vi "Autonomous Independent.vi"   [LabVIEW 2015]
doc: "This VI is called when autonomous begins, and will automatically be terminated when autonomous ends. You can carry out timed or sensor driven robot movement independently without needing to return to the caller."
uses:
  <vilib>/Rock Robotics/WPI/Utilities/WPI_GetSetVariantRefNum.vi
  <vilib>/Rock Robotics/Network Tables/NT Read String.vi
  <vilib>/Rock Robotics/Network Tables/NT Write Numeric Array.vi
panel:
  # "Be sure to right-click and choose Data Operations>>Make Current Value default if you want to save the array values with the VI"
types:
  T1 = typedef "WPI_JoystickDevRef.ctl" = cluster{"Device":T2}
  T2 = typedef "WPI_JoystickDeviceEnum.ctl" = enum16{"USB 0", "USB 1", "USB 2", "USB 3", "USB 4", "USB 5"}
  T3 = typedef "WPI_ServoDeviceRef.ctl" = cluster{"DeviceStatus":errorcluster, "PWM Channel":T4, "DeadBand":T5}
  T4 = typedef "FPGA_DIOPWMChannel.ctl" = enum8{"PWM 0", "PWM 1", "PWM 2", "PWM 3", "PWM 4", "PWM 5", "PWM 6", "PWM 7", "PWM 8", "PWM 9", "PWM MXP 0", "PWM MXP 1", "PWM MXP 2", "PWM MXP 3", "PWM MXP 4", "PWM MXP 5", "PWM MXP 6", "PWM MXP 7", "PWM MXP 8", "PWM MXP 9", "Invalid"}
  T5 = typedef "WPI_PWMDeadband.ctl" = cluster{"Name":string, "maxPositivePwm":i32, "minPositivePwm":i32, "centerPwm":i32, "maxNegativePwm":i32, "minNegativePwm":i32, "angularRange":u16}
  T6 = typedef "WPI_DigitalInputDevRef.ctl" = cluster{"DevStatus":errorcluster, "DIO Channel":T7}
  T7 = typedef "FPGA_DIOChannel.ctl" = enum8{"DIO 0", "DIO 1", "DIO 2", "DIO 3", "DIO 4", "DIO 5", "DIO 6", "DIO 7", "DIO 8", "DIO 9", "DIO MXP 0", "DIO MXP 1", "DIO MXP 2", "DIO MXP 3", "DIO MXP 4", "DIO MXP 5", "DIO MXP 6", "DIO MXP 7", "DIO MXP 8", "DIO MXP 9", "DIO MXP 10", "DIO MXP 11", "DIO MXP 12", "DIO MXP 13", "DIO MXP 14", "DIO MXP 15", "Invalid"}
  T8 = typedef "WPI_MotorControlDeviceRef.ctl" = cluster{"DeviceStatus":errorcluster, "Type":T9, "PWM":cluster{"PWM Channel":T4, "DeadBand":T5}, "CAN":cluster{"Device Number":u8, "Control Mode":T10, "Semaphore":T11, "Max Vout":dbl, "TalonSRX Control Mode":T12}, "Invert":bool}
  T9 = typedef "WPI_MotorControlType.ctl" = enum16{"PWM", "CAN", "CANTalonSRX"}
  T10 = typedef "WPI_CANJaguar_ControlMode.ctl" = enum8{"Percent VBus", "Current", "Speed", "Position", "Voltage"}
  T11 = typedef "Semaphore RefNum" = refnum<k1>
  T12 = typedef "WPI_CANTalonSRX_APIControlMode.ctl" = enum8{"Percent VBus", "Speed", "Position", "Slave", "Unchanged / Invalid", "Voltage Compensation", "Current", "Motion Profile"}
  T13 = typedef "WPI_RobotDriveDevRef.ctl" = cluster{"DevStatus":errorcluster, "Motors[]":T8[], "Square Inputs":bool, "Max Output":dbl}
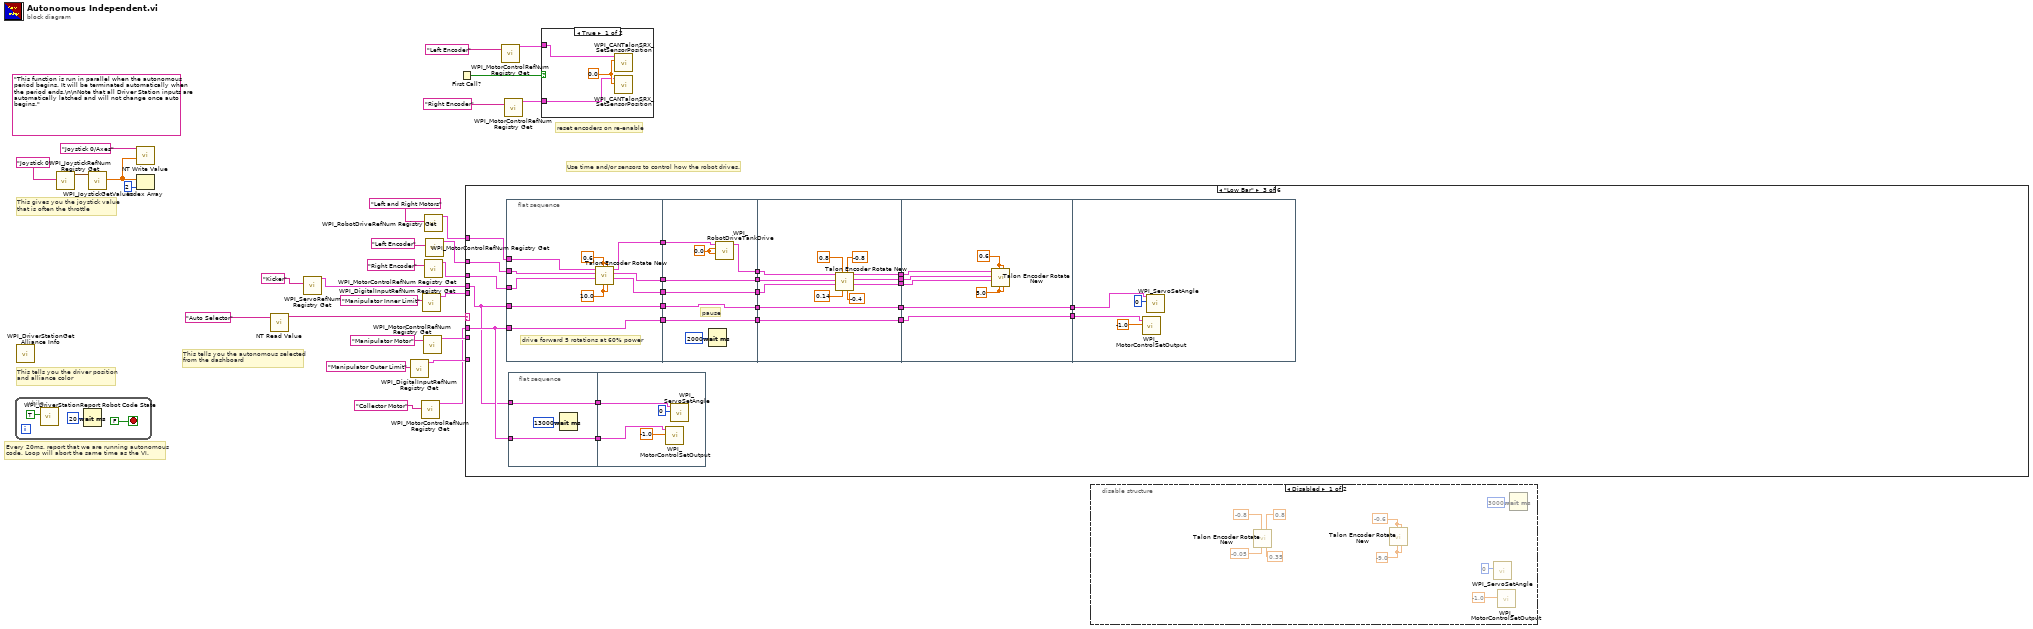
[diagram p0: block diagram]
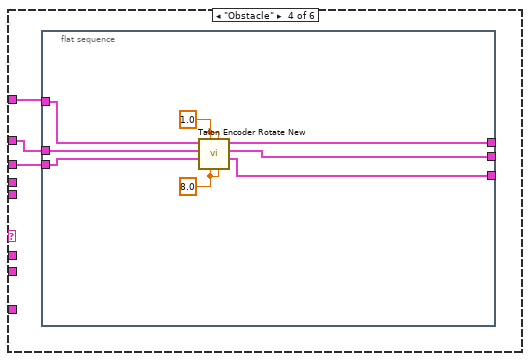
[diagram p6: hidden frame]
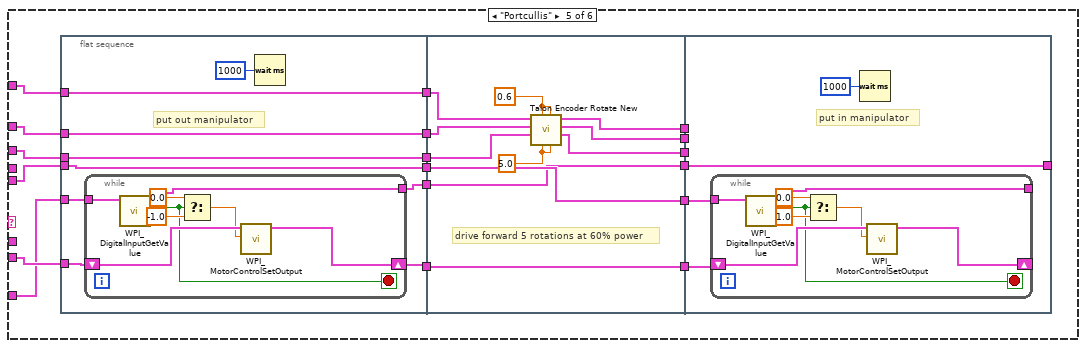
[diagram p7: hidden frame]
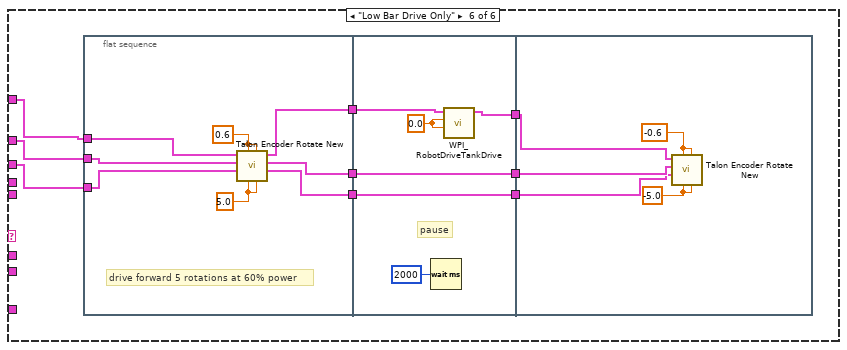
[diagram p8: hidden frame]
diagram:
  (unwired) "This function is run in parallel when the autonomous period begins. It will be terminated automatically when the period ends.\n\nNote that all Driver Station inputs are automatically latched and will not change once auto begins."
  # "reset encoders on re-enable"
  # "This tells you the autonomous selected\nfrom the dashboard"
  # "Every 20ms, report that we are running autonomous\ncode. Loop will abort the same time as the VI."
  # "This gives you the joystick value\nthat is often the throttle"
  # "Use time and/or sensors to control how the robot drives."
  # "This tells you the driver position\nand alliance color"
  n1 = while {
    stop <- FALSE stop-if-true
    n2 = call <vilib>:"WPI_DriverStationReport Robot Code State.vi"("Autonomous"=TRUE) -> ()  [unwired: 10 in, 1 out]
    n3 = Wait (ms)(milliseconds to wait=u32 20) -> ()  [unwired: 1 out]
  }
  n4 = call <vilib>:"WPI_DriverStationGet Alliance Info.vi"() -> ()  [unwired: 12 out]
  n5 = call <vilib>:"WPI_JoystickRefNum Registry Get.vi"("refnum name"="Joystick 0") -> ("JoystickDevRef"=w27:T1)  [unwired: 1 in, 9 out]
  n6 = call <vilib>:"WPI_JoystickGetValues.vi"("JoystickDevRef"=w27) -> ("Axes"=w23:dbl[])  [unwired: 6 in, 4 out]
  n7 = call-poly <vilib>:"NT Write Value.vi"("Numeric Array"=w23, "Name"="Joystick 0/Axes") -> ()  [unwired: 9 in, 1 out]
  n8 = Index Array(array=w23, index=2) -> ()  [unwired: 1 out]
  n9 = call-poly <vilib>:"NT Read Value.vi"("Name"="Auto Selector") -> ("String"=w24:string)  [unwired: 9 in, 1 out]
  n10 = call <vilib>:"WPI_ServoRefNum Registry Get.vi"("refnum name"="Kicker") -> ("ServoDeviceRef"=w1:T3)  [unwired: 9 in, 1 out]
  n11 = call <vilib>:"WPI_DigitalInputRefNum Registry Get.vi"("refnum name"="Manipulator Outer Limit") -> ("DigitalInputDevRef"=w7:T6)  [unwired: 9 in, 1 out]
  n12 = call <vilib>:"WPI_MotorControlRefNum Registry Get.vi"("refnum name"="Collector Motor") -> ("MotorControlDevRef"=w3:T8)  [unwired: 9 in, 1 out]
  n13 = call <vilib>:"WPI_DigitalInputRefNum Registry Get.vi"("refnum name"="Manipulator Inner Limit") -> ("DigitalInputDevRef"=w5:T6)  [unwired: 9 in, 1 out]
  n14 = call <vilib>:"WPI_MotorControlRefNum Registry Get.vi"("refnum name"="Manipulator Motor") -> ("MotorControlDevRef"=w9:T8)  [unwired: 9 in, 1 out]
  n15 = call <vilib>:"WPI_RobotDriveRefNum Registry Get.vi"("refnum name"="Left and Right Motors") -> ("RobotDriveDevRef"=w13:T13)  [unwired: 1 in, 9 out]
  n16 = call <vilib>:"WPI_MotorControlRefNum Registry Get.vi"("refnum name"="Right Encoder") -> ("MotorControlDevRef"=w12:T8)  [unwired: 9 in, 1 out]
  n17 = call <vilib>:"WPI_MotorControlRefNum Registry Get.vi"("refnum name"="Left Encoder") -> ("MotorControlDevRef"=w11:T8)  [unwired: 9 in, 1 out]
  n18 = First Call?() -> (First Call?: T/F=w21:bool)
  n19 = case shown="\"Low Bar\"" w24 {
    tunnel: w13 -> [_ _ w55 w106 w132 w178]
    tunnel: w12 -> [_ _ w53 w104 w130 w176]
    tunnel: w11 -> [_ _ w54 w105 w131 w177]
    tunnel: w9 -> [_ _ _ _ w129 _]
    tunnel: w7 -> [_ _ _ _ w128 _]
    tunnel: w5 -> [_ _ _ _ w123 _]
    tunnel: w3 -> [_ _ w34 _ _ _]
    tunnel: w1 -> [_ _ w32 _ _ _]
    frame "None", Default {
    }
    frame "Teeter Totter" {
    }
    frame "Low Bar" {
      n20 = flat-sequence {
        tunnel: w55 -> [w72]
        tunnel: w54 -> [w71]
        tunnel: w53 -> [w70]
        tunnel: [w69] -> w51
        tunnel: [w66] -> w49
        tunnel: [w65] -> w47
        tunnel: [w64] -> w41
        tunnel: w34 -> [w64]
        tunnel: w32 -> [w63]
        tunnel: [w63] -> w38
        tunnel: [w80] -> w52
        tunnel: w51 -> [w77]
        tunnel: [w76] -> w50
        tunnel: w49 -> [w76]
        tunnel: [w75] -> w48
        tunnel: w47 -> [w75]
        tunnel: [w74] -> w42
        tunnel: w41 -> [w74]
        tunnel: [w73] -> w39
        tunnel: w38 -> [w73]
        tunnel: w52 -> [w92]
        tunnel: w50 -> [w91]
        tunnel: w48 -> [w90]
        tunnel: [w89] -> w46
        tunnel: [w88] -> w45
        tunnel: [w87] -> w44
        tunnel: [w82] -> w43
        tunnel: w42 -> [w82]
        tunnel: [w81] -> w40
        tunnel: w39 -> [w81]
        tunnel: w46 -> [w98]
        tunnel: w45 -> [w97]
        tunnel: w44 -> [w96]
        tunnel: w43 -> [w93]
        tunnel: w40 -> [w94]
        tunnel: [w94] -> w37
        tunnel: [w93] -> w36
        tunnel: w37 -> [w101]
        tunnel: w36 -> [w100]
        frame #0 {
          w67 = 10.0 ("Rotations")
          w68 = 0.6 ("Speed")
          # "drive forward 5 rotations at 60% power"
          n21 = call "Talon Encoder Rotate New.vi"("Right Rotations"=w67, "Right Speed"=w68, "Left Rotations"=w67, "Left Speed"=w68, "RightEncoderMotorRef"=w70, "LeftEncoderMotorRef"=w71, "RobotDriveDevRef"=w72) -> ("RightEncoderMotorRef"=w65:T8, "LeftEncoderMotorRef"=w66:T8, "RobotDriveDevRef"=w69:T13)  [unwired: 2 in]
        }
        frame #1 {
          w79 = 0.0 ("Left axis value")
          # "pause"
          n22 = Wait (ms)(milliseconds to wait=u32 2000) -> ()  [unwired: 1 out]
          n23 = call <vilib>:"WPI_RobotDriveTankDrive.vi"("Right axis value"=w79, "Left axis value"=w79, "RobotDriveDevRef"=w77) -> ("RobotDriveDevRef"=w80:T13)  [unwired: 6 in, 2 out]
        }
        frame #2 {
          n24 = call "Talon Encoder Rotate New.vi"("Right Rotations"=-0.4, "Right Speed"=-0.8, "Left Rotations"=0.14, "Left Speed"=0.8, "RightEncoderMotorRef"=w90, "LeftEncoderMotorRef"=w91, "RobotDriveDevRef"=w92) -> ("RightEncoderMotorRef"=w87:T8, "LeftEncoderMotorRef"=w88:T8, "RobotDriveDevRef"=w89:T13)  [unwired: 2 in]
        }
        frame #3 {
          w95 = 5.0 ("Left Rotations")
          w99 = 0.6 ("Speed")
          n25 = call "Talon Encoder Rotate New.vi"("Right Rotations"=w95, "Right Speed"=w99, "Left Rotations"=w95, "Left Speed"=w99, "RightEncoderMotorRef"=w96, "LeftEncoderMotorRef"=w97, "RobotDriveDevRef"=w98) -> ()  [unwired: 2 in, 3 out]
        }
        frame #4 {
          n26 = call <vilib>:"WPI_MotorControlSetOutput.vi"("Output"=-1.0, "MotorControlDevRef"=w100) -> ()  [unwired: 7 in, 3 out]
          n27 = call <vilib>:"WPI_ServoSetAngle.vi"("Angle"=0, "ServoDeviceRef"=w101) -> ()  [unwired: 8 in, 2 out]
        }
      }
      n28 = flat-sequence {
        tunnel: [w57] -> w35
        tunnel: w34 -> [w57]
        tunnel: [w56] -> w33
        tunnel: w32 -> [w56]
        tunnel: w35 -> [w60]
        tunnel: w33 -> [w59]
        frame #0 {
          n29 = Wait (ms)(milliseconds to wait=u32 13000) -> ()  [unwired: 1 out]
        }
        frame #1 {
          n30 = call <vilib>:"WPI_MotorControlSetOutput.vi"("Output"=-1.0, "MotorControlDevRef"=w60) -> ()  [unwired: 7 in, 3 out]
          n31 = call <vilib>:"WPI_ServoSetAngle.vi"("Angle"=0, "ServoDeviceRef"=w59) -> ()  [unwired: 8 in, 2 out]
        }
      }
    }
    frame "Obstacle" {
      n32 = flat-sequence {
        tunnel: w106 -> [w114]
        tunnel: w105 -> [w113]
        tunnel: w104 -> [w112]
        tunnel: [w109] -> _
        tunnel: [w108] -> _
        tunnel: [w107] -> _
        frame #0 {
          w110 = 8.0 ("Rotations")
          w111 = 1.0 ("Speed")
          n33 = call "Talon Encoder Rotate New.vi"("Right Rotations"=w110, "Right Speed"=w111, "Left Rotations"=w110, "Left Speed"=w111, "RightEncoderMotorRef"=w112, "LeftEncoderMotorRef"=w113, "RobotDriveDevRef"=w114) -> ("RightEncoderMotorRef"=w107:T8, "LeftEncoderMotorRef"=w108:T8, "RobotDriveDevRef"=w109:T13)  [unwired: 2 in]
        }
      }
    }
    frame "Portcullis" {
      n34 = flat-sequence {
        tunnel: w129 -> [w138]
        tunnel: w132 -> [w139]
        tunnel: w130 -> [w140]
        tunnel: w131 -> [w141]
        tunnel: [w141] -> w120
        tunnel: [w140] -> w119
        tunnel: [w139] -> w118
        tunnel: [w137] -> w117
        tunnel: w128 -> [w136]
        tunnel: w123 -> [w134]
        tunnel: [w134] -> w116
        tunnel: [w133] -> w115
        tunnel: w120 -> [w158]
        tunnel: w119 -> [w157]
        tunnel: w118 -> [w159]
        tunnel: w117 -> [w160]
        tunnel: [w160] -> w127
        tunnel: [w154] -> w126
        tunnel: [w153] -> w125
        tunnel: [w152] -> w124
        tunnel: [w151] -> w122
        tunnel: w116 -> [w151]
        tunnel: w115 -> [w150]
        tunnel: [w150] -> w121
        tunnel: w127 -> [w164]
        tunnel: w126 -> [_]
        tunnel: w125 -> [_]
        tunnel: w124 -> [_]
        tunnel: w122 -> [w163]
        tunnel: w121 -> [w161]
        tunnel: [w161] -> _
        frame #0 {
          # "put out manipulator"
          n35 = while {
            shift-right: [w148] -> w137
            shift-left: w138 -> [w149]
            tunnel: w136 -> [w147]
            tunnel: [w142] -> w133
            stop <- w143 stop-if-true
            n36 = call <vilib>:"WPI_DigitalInputGetValue.vi"("DigitalInputDevRef"=w147) -> ("Value"=w143:bool, "DigitalInputDevRef"=w142:T6)  [unwired: 8 in, 1 out]
            n37 = Select(t=0.0, s=w143, f=-1.0) -> (s? t:f=w144:dbl)
            n38 = call <vilib>:"WPI_MotorControlSetOutput.vi"("Output"=w144, "MotorControlDevRef"=w149) -> ("MotorControlDevRef"=w148:T8)  [unwired: 7 in, 2 out]
          }
          n39 = Wait (ms)(milliseconds to wait=u32 1000) -> ()  [unwired: 1 out]
        }
        frame #1 {
          w156 = 5.0 ("Left Rotationos")
          w155 = 0.6 ("Speed")
          # "drive forward 5 rotations at 60% power"
          n40 = call "Talon Encoder Rotate New.vi"("Right Rotations"=w156, "Right Speed"=w155, "Left Rotations"=w156, "Left Speed"=w155, "RightEncoderMotorRef"=w157, "LeftEncoderMotorRef"=w158, "RobotDriveDevRef"=w159) -> ("RightEncoderMotorRef"=w152:T8, "LeftEncoderMotorRef"=w153:T8, "RobotDriveDevRef"=w154:T13)  [unwired: 2 in]
        }
        frame #2 {
          # "put in manipulator"
          n41 = while {
            shift-right: [w171] -> _
            shift-left: w164 -> [w172]
            tunnel: w163 -> [w170]
            tunnel: [w165] -> _
            stop <- w166 stop-if-true
            n42 = call <vilib>:"WPI_DigitalInputGetValue.vi"("DigitalInputDevRef"=w170) -> ("Value"=w166:bool, "DigitalInputDevRef"=w165:T6)  [unwired: 8 in, 1 out]
            n43 = Select(t=0.0, s=w166, f=1.0) -> (s? t:f=w167:dbl)
            n44 = call <vilib>:"WPI_MotorControlSetOutput.vi"("Output"=w167, "MotorControlDevRef"=w172) -> ("MotorControlDevRef"=w171:T8)  [unwired: 7 in, 2 out]
          }
          n45 = Wait (ms)(milliseconds to wait=u32 1000) -> ()  [unwired: 1 out]
        }
      }
    }
    frame "Low Bar Drive Only" {
      n46 = flat-sequence {
        tunnel: w178 -> [w189]
        tunnel: w177 -> [w188]
        tunnel: w176 -> [w187]
        tunnel: [w186] -> w181
        tunnel: [w183] -> w180
        tunnel: [w182] -> w179
        tunnel: w181 -> [w193]
        tunnel: w180 -> [w191]
        tunnel: w179 -> [w190]
        tunnel: [w192] -> w175
        tunnel: [w191] -> w174
        tunnel: [w190] -> w173
        tunnel: w175 -> [w198]
        tunnel: w174 -> [w197]
        tunnel: w173 -> [w196]
        frame #0 {
          w184 = 5.0 ("Rotations")
          w185 = 0.6 ("Speed")
          # "drive forward 5 rotations at 60% power"
          n47 = call "Talon Encoder Rotate New.vi"("Right Rotations"=w184, "Right Speed"=w185, "Left Rotations"=w184, "Left Speed"=w185, "RightEncoderMotorRef"=w187, "LeftEncoderMotorRef"=w188, "RobotDriveDevRef"=w189) -> ("RightEncoderMotorRef"=w182:T8, "LeftEncoderMotorRef"=w183:T8, "RobotDriveDevRef"=w186:T13)  [unwired: 2 in]
        }
        frame #1 {
          w195 = 0.0 ("Left axis value")
          # "pause"
          n48 = Wait (ms)(milliseconds to wait=u32 2000) -> ()  [unwired: 1 out]
          n49 = call <vilib>:"WPI_RobotDriveTankDrive.vi"("Right axis value"=w195, "Left axis value"=w195, "RobotDriveDevRef"=w193) -> ("RobotDriveDevRef"=w192:T13)  [unwired: 6 in, 2 out]
        }
        frame #2 {
          w199 = -5.0 ("Left Rotations")
          w200 = -0.6 ("Speed")
          n50 = call "Talon Encoder Rotate New.vi"("Right Rotations"=w199, "Right Speed"=w200, "Left Rotations"=w199, "Left Speed"=w200, "RightEncoderMotorRef"=w196, "LeftEncoderMotorRef"=w197, "RobotDriveDevRef"=w198) -> ()  [unwired: 2 in, 3 out]
        }
      }
    }
  }
  n51 = call <vilib>:"WPI_MotorControlRefNum Registry Get.vi"("refnum name"="Left Encoder") -> ("MotorControlDevRef"=w19:T8)  [unwired: 9 in, 1 out]
  n52 = call <vilib>:"WPI_MotorControlRefNum Registry Get.vi"("refnum name"="Right Encoder") -> ("MotorControlDevRef"=w18:T8)  [unwired: 9 in, 1 out]
  n53 = case shown="True" w21 {
    tunnel: w19 -> [w202 _]
    tunnel: w18 -> [w201 _]
    frame True {
      w203 = 0.0
      n54 = call <vilib>:"WPI_CANTalonSRX_SetSensorPosition.vi"("New Sensor Position"=w203, "CAN Talon SRX Ref"=w202) -> ()  [unwired: 8 in, 2 out]
      n55 = call <vilib>:"WPI_CANTalonSRX_SetSensorPosition.vi"("New Sensor Position"=w203, "CAN Talon SRX Ref"=w201) -> ()  [unwired: 8 in, 2 out]
    }
    frame False {
    }
  }
  n56 = disable-structure shown="Disabled" {
    frame Disabled {
      w209 = -9.0 ("Rotations")
      w210 = -0.6 ("Speed")
      n57 = call "Talon Encoder Rotate New.vi"("Right Rotations"=0.35, "Right Speed"=0.8, "Left Rotations"=-0.05, "Left Speed"=-0.8) -> ()  [unwired: 5 in, 3 out]
      n58 = call "Talon Encoder Rotate New.vi"("Right Rotations"=w209, "Right Speed"=w210, "Left Rotations"=w209, "Left Speed"=w210) -> ()  [unwired: 5 in, 3 out]
      n59 = call <vilib>:"WPI_ServoSetAngle.vi"("Angle"=0) -> ("ServoDeviceRef"=w205:T3)  [unwired: 8 in, 2 out]
      n60 = call <vilib>:"WPI_MotorControlSetOutput.vi"("Output"=-1.0) -> ("MotorControlDevRef"=w208:T8)  [unwired: 7 in, 3 out]
      n61 = Wait (ms)(milliseconds to wait=u32 3000) -> ()  [unwired: 1 out]
    }
    frame Enabled {
    }
  }
